vi "LVClass_CameraSet GetGenericParameterRealValue.vi"(0 "CameraSet.lvclass":refnum<class "CameraSet.lvclass">, 5 "parameter_name":string, 7 "DefaultFactorySet":bool, 11 "error in (no error)":errorcluster) -> (4 "CameraSet.lvclass":refnum<class "CameraSet.lvclass">, 6 "Value":dbl, 15 "error out":errorcluster)   [LabVIEW 2020, in "CameraSet.lvclass"]
doc: "Camera parameter value getter for parameter of type float.\n\n<B>camera_setIn</B> : CameraSet object.\n<B>camera_setOut</B> : CameraSet object.\n<B>parameter_name</B> : Parameter name.\n<B>value</B> : Parameter value."
uses:
  CameraSet.lvclass
  CameraSet.lvclass/CameraSet.ctl
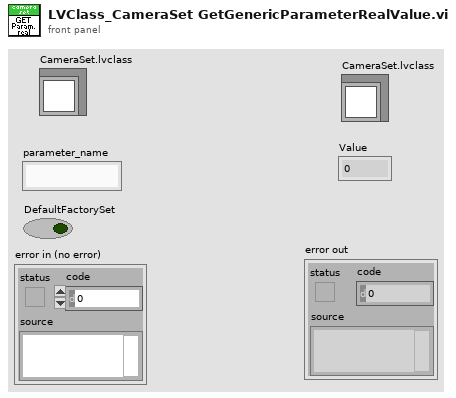
[diagram p1: front panel]
types:
  T1 = typedef "ClassID.ctl" = i64
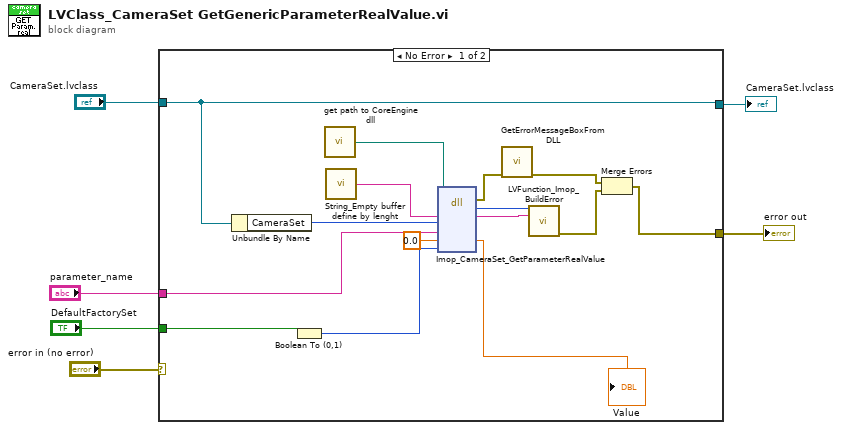
[diagram p0: block diagram]
diagram:
  n1 = case shown="No Error" "error in (no error)" {
    selector: "error in (no error)" -> [_ w22]
    tunnel: "CameraSet.lvclass" -> [w14 w23]
    tunnel: [w14 w23] -> w4
    tunnel: [w11 w22] -> w3
    tunnel: "DefaultFactorySet" -> [w9 _]
    tunnel: "parameter_name" -> [w8 _]
    frame No Error {
      n2 = Unbundle By Name(w14) -> ("CameraSet"=w13:T1)
      n3 = Boolean To (0,1)(Boolean=w9) -> (0, 1=w7:i16)
      n4 = call "get path to CoreEngine dll.vi"() -> ("path to c_interface_vc100.dll"=w17:path)  [unwired: 12 in, 3 out]
      n5 = call "String_Empty buffer define by lenght.vi"() -> ("Empty buffer"=w19:string)  [unwired: 1 in]
      n6 = dll-call lib="D:/2_trunk/Soft_haso/ImOpCoreEngine4_LV2011/DLLs/ImopEngine4_vc100.dll" fn="Imop_CameraSet_GetParameterRealValue"(path in=w17, "message"=w19, "objet"=w13, "parameter_name"=w8, "Value"=0.0 ("min"), "DefaultFactorySet"=w7) -> (error out=w16:errorcluster, "return type"=w21:i32, "message"=w20:string, "Value"=→"Value":dbl)  [unwired: 5 in, 1 out]
      n7 = call "GetErrorMessageBoxFromDLL.vi"("error IN"=w16) -> ("error OUT"=w10:errorcluster)  [unwired: 10 in]
      n8 = call "LVFunction_Imop_BuildError.vi"("code"=w21, "String to Prepend to source (\"\")"=w20) -> ("error out"=w12:errorcluster)  [unwired: 13 in]
      n9 = Merge Errors(w10, w12) -> (w11:errorcluster)
    }
    frame Error {
    }
  }
  "CameraSet.lvclass" <- w4
  "error out" <- w3
